vi "CheckHandle.vi"(6 "Array":T1(array[cluster]), 8 "Error In":errorcluster, 11 "Handle In":string) -> (0 "Error Out":errorcluster, 1 "Instrument Handle":refnum<k15>, 2 "Handle Connected?":bool, 3 "Handle Out":string)   [LabVIEW 2018, in "AcPwrPlugins.lvlib" / "ChromaAcLoad.lvclass"]
doc: "This VI checks to see if the input handle is already connected."
uses:
  ChromaAcLoad.lvclass
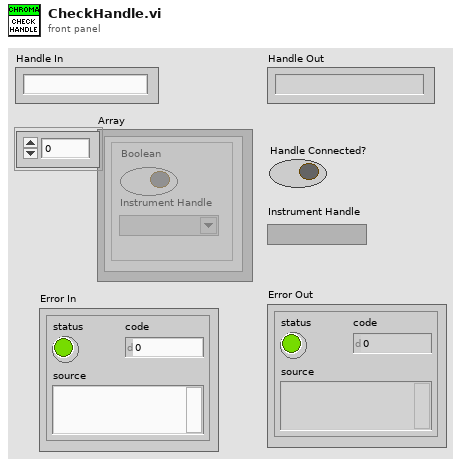
[diagram p1: front panel]
types:
  T1 = cluster{"Boolean":bool, "Instrument Handle":refnum<k15>}[]
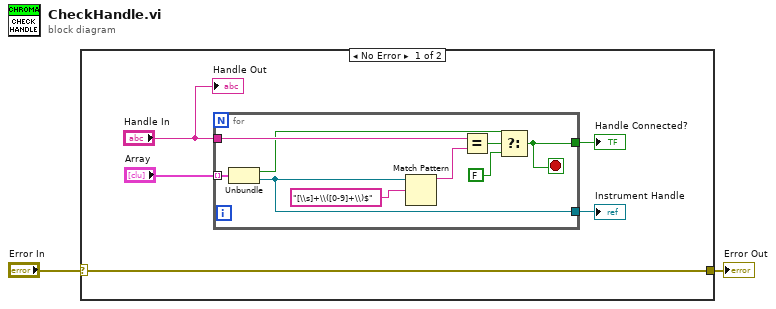
[diagram p0: block diagram]
diagram:
  n1 = case shown="No Error" "Error In" {
    selector: "Error In" -> [w5 w17]
    tunnel: [w5 w17] -> w1
    frame No Error {
      n2 = for {
        tunnel: "Handle In" -> [w16]
        tunnel: [w14] -> w6
        tunnel: "Array" -> [w10] mode=indexing
        tunnel: [w8] -> w3
        stop <- w14 stop-if-true
        n3 = Unbundle(w10) -> ("Boolean"=w9:bool, "Instrument Handle"=w8:refnum<k15>)
        n4 = Match Pattern(string=w8, regular expression="[\\s]+\\([0-9]+\\)$") -> (before substring=w12:string)  [unwired: 1 in, 3 out]
        n5 = Equal?(x=w16, y=w12) -> (x = y?=w15:bool)
        n6 = Select(t=w9, s=w15, f=FALSE) -> (s? t:f=w14:bool)
      }
      "Handle Connected?" <- w6
      "Instrument Handle" <- w3
      "Handle Out" <- "Handle In"
    }
    frame Error {
    }
  }
  "Error Out" <- w1
